vi "ObtainQueue.vi"(8 "error in (no error)":errorcluster, 10 "# Priority Levels (5)":i32=5) -> (0 "error out":errorcluster, 3 "PriorityQueue out":refnum<class "PriorityQueue.lvclass">)   [LabVIEW 2019, in "PriorityQueue.lvclass"]
doc: "Creates a PriorityQueue object with the specified number of available priority levels.\n\nPriority levels are numbered from 0 to n-1, with level 0 being the highest priority and level n-1 being the lowest priority."
uses:
  PriorityQueue.lvclass
  PriorityQueue.lvclass/PriorityQueue.ctl
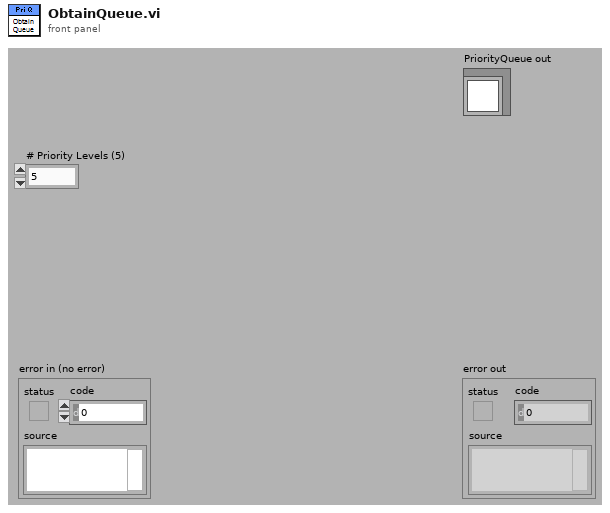
[diagram p1: front panel]
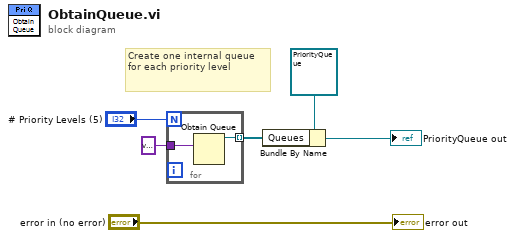
[diagram p0: block diagram]
diagram:
  # "Create one internal queue for each priority level"
  n1 = for {
    N: "# Priority Levels (5)" -> [_]
    tunnel: variant ("element data type") -> [w8]
    tunnel: [w7] -> w2 mode=indexing
    n2 = Obtain Queue(element data type=w8) -> (queue out=w7:refnum<queue>)  [unwired: 4 in, 2 out]
  }
  n3 = Bundle By Name(cluster=refnum<class "PriorityQueue.lvclass"> refnum ("PriorityQueue in"), "Queues"=w2) -> (→"PriorityQueue out":refnum<class "PriorityQueue.lvclass">)
  "error out" <- "error in (no error)"
